vi "FG WaypointList.vi"(1 "FG Action (Read)":T3, 2 "Local Waypoint List in":T1[](array[typedef])) -> (0 "Local Waypoint List out":T1[](array[typedef]))   [LabVIEW 2009]
uses:
  cRIO/Functional Global Variables/Actions for FG's.ctl
  ElementRec.ctl
  LocalWaypointRec.ctl
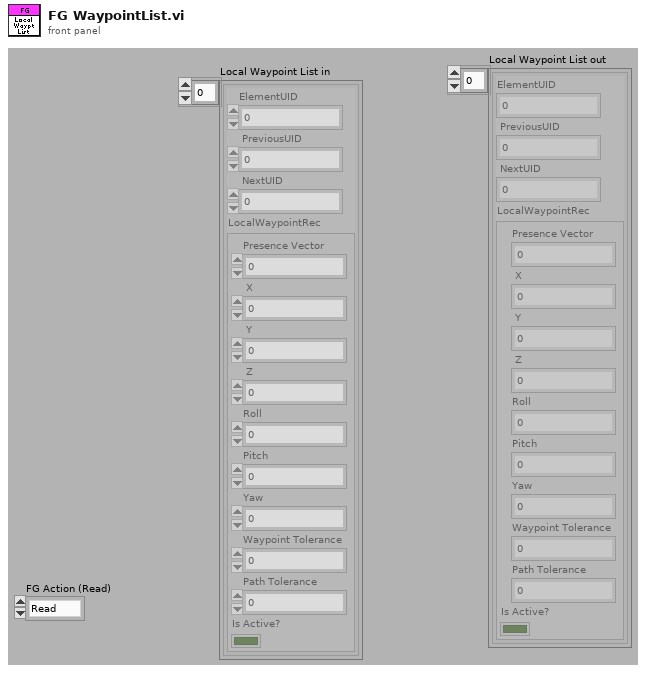
[diagram p1: front panel]
types:
  T1 = typedef "ElementRec.ctl" = cluster{"ElementUID":u16, " PreviousUID":u16, " NextUID":u16, "LocalWaypointRec":T2}
  T2 = typedef "LocalWaypointRec.ctl" = cluster{"Presence Vector":u8, " X":dbl, " Y":dbl, " Z":dbl, "Roll":dbl, "Pitch":dbl, "Yaw":dbl, "Waypoint Tolerance":dbl, "Path Tolerance":dbl, "Is Active?":bool}
  T3 = typedef "Actions for FG's.ctl" = enum16{"Read", "Write"}
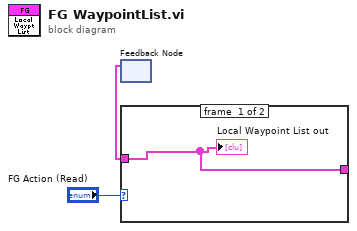
[diagram p0: block diagram]
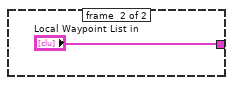
[diagram p2: hidden frame]
diagram:
  n1 = feedback #1() -> (w1:T1[])  [unwired: 1 in]
  n2 = case shown="\"Write\"" "FG Action (Read)" {
    tunnel: [w4 "Local Waypoint List in"] -> w3
    tunnel: w1 -> [w4 _]
    frame #0 {
      "Local Waypoint List out" <- w4
    }
    frame #1 {
    }
  }
